vi "zero_detection_simulation.vi"() -> ()   [LabVIEW 2021]
uses:
  <vilib>/Platform/TimedLoop/XDataNode/timing_clust.ctl
  <vilib>/Platform/TimedLoop/XDataNode/nitl_modes.ctl
  <vilib>/Platform/TimedLoop/XDataNode/wakeup.ctl
  <vilib>/Platform/TimedLoop/XDataNode/XDataNode.xnode
  <vilib>/Platform/TimedLoop/XDataNode/XDNodeRunTimeDep.lvlib
panel:
  in  "stop 2":bool
  out "output":dbl(slide) scale=-1.0..1.0
  in  "fractional index or x":dbl(slide) scale=0.0..1.0
  out "size(s)":i32
  in  "sin wave":dbl
  in  "memory down sampling rate":i32
  in  "zero detect down sampling rate":i32
  out "Waveform Graph":dbl[](graph)
  out "appended array":dbl[](array[numeric])
  out "Disturbance(x)":dbl(graph)
  in  "stop":bool
  # "Disturbance"
  # "Online Segmentaion"
  # "Phase"
  # "Memory"
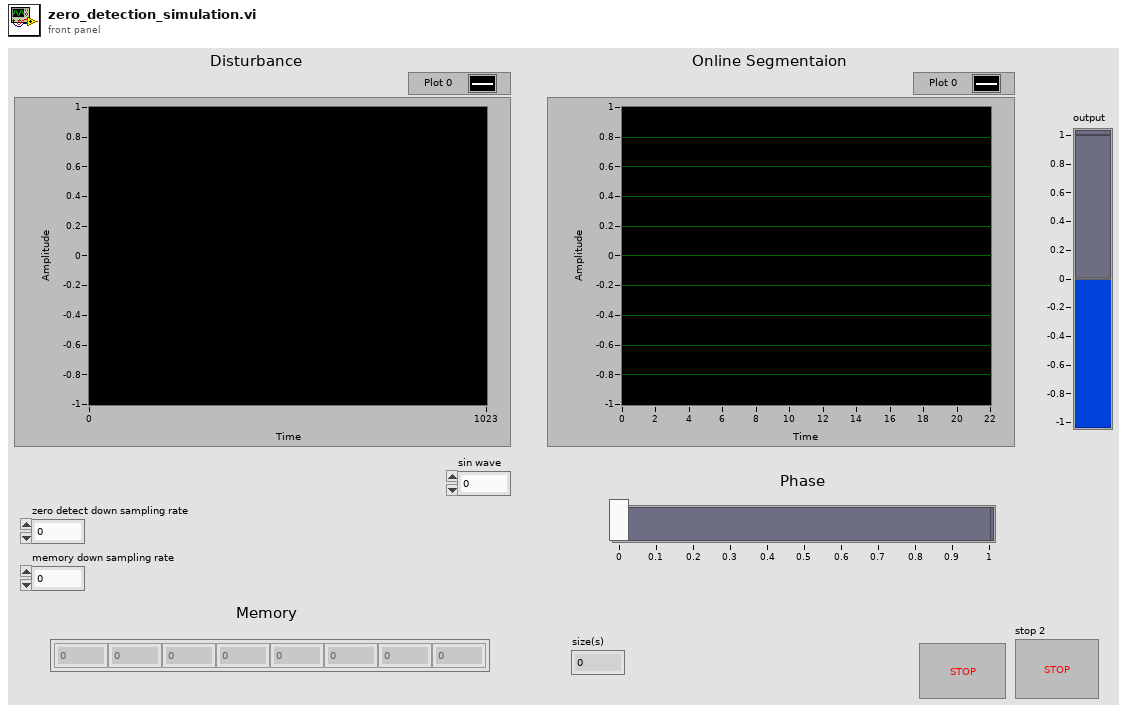
[diagram p1: front panel]
types:
  T1 = typedef "XDNodeRunTimeDep.lvlib/timing_clust.ctl" = cluster{"Expected End [f-1]":u64, "Actual End [f-1]":u64, "Finished Late? [f-1]":bool, "Expected End [i-1]":u64, "Actual End [i-1]":u64, "Finished Late? [i-1]":bool, "Expected Start [i]":u64, "Actual Start [i]":u64, "Expected Start [f]":u64, "Actual Start [f]":u64, "Source Name":string, "Structure Name":string, "Period":i64, "Deadline":i64, "Offset":i64, "Start":i64, "Priority":i32, "Timeout":i32, "Mode":T2, "Wakeup Reason":T3, "Error":errorcluster, "Source Type":string, "Secondary Source Type":string, "Global End Time":u64, "Global Start Time":u64, "Frame Duration":u64, "Iteration Duration":u64, "Assigned CPU":i32, "I/O Scan Engine Mode":u32}
  T2 = typedef "XDNodeRunTimeDep.lvlib/nitl_modes.ctl" = enum32{"No Change", "Process missed periods, maintain original phase", "Discard missed periods, maintain original phase", "Process missed periods, ignore original phase", "Discard missed periods, ignore original phase"}
  T3 = typedef "XDNodeRunTimeDep.lvlib/wakeup.ctl" = enum32{"Normal", "Aborted", "Asynchronous wakeup", "Timing source error", "Timed loop error", "Timeout"}
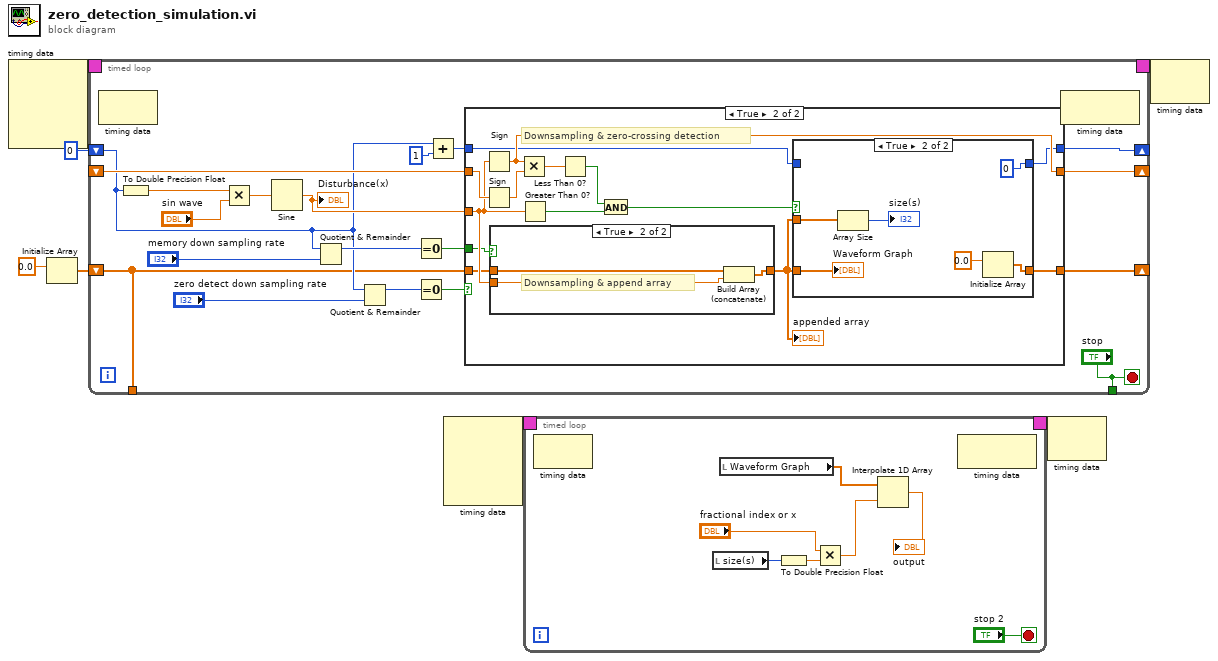
[diagram p0: block diagram]
diagram:
  n1 = node-c288() -> (w4:T1)  [unwired: 4 in]
  n2 = Initialize Array(0.0 ("element")) -> (w5:dbl[])  [unwired: 1 in]
  n3 = timed-loop {
    shift-right: [w23] -> _
    shift-left: _ -> [w22]
    shift-right: [w10] -> _
    shift-left: w5 -> [w9]
    shift-right: [w15] -> _
    shift-left: 0 -> [w16]
    timing: w4 -> [_]
    timing-out: [_] -> w3
    tunnel: [w9] -> _
    tunnel: ["stop"] -> _
    stop <- "stop" stop-if-true
    n4 = node-c288() -> ()  [unwired: 1 in, 1 out]
    n5 = To Double Precision Float(number=w16) -> (double precision float=w26:dbl)
    n6 = Multiply(x=w26, y="sin wave") -> (x*y=w21:dbl)
    n7 = Sine(x=w21) -> (sin(x)=w20:dbl)
    "Disturbance(x)" <- w20
    n8 = Quotient & Remainder(x=w16, y="memory down sampling rate") -> (x-y*floor(x/y)=w19:i32)  [unwired: 1 out]
    n9 = Quotient & Remainder(x=w16, y="zero detect down sampling rate") -> (x-y*floor(x/y)=w25:i32)  [unwired: 1 out]
    n10 = Equal To 0?(x=w19) -> (x = 0?=w18:bool)
    n11 = Equal To 0?(x=w25) -> (x = 0?=w24:bool)
    n12 = Add(x=w16, y=1) -> (x+y=w14:i32)
    n13 = case shown="True" w24 {
      tunnel: w20 -> [_ w40]
      tunnel: [w31 w43] -> w23
      tunnel: w22 -> [w31 w42]
      tunnel: [w30 w41] -> w10
      tunnel: w9 -> [w30 w34]
      tunnel: w18 -> [_ w32]
      tunnel: [w29 w36] -> w15
      tunnel: w14 -> [w29 w35]
      frame False {
      }
      frame True {
        # "Downsampling & zero-crossing detection"
        n14 = Sign(1:w40) -> (0:w43:dbl)
        n15 = Sign(1:w42) -> (0:w44:dbl)
        n16 = case shown="True" w32 {
          tunnel: w34 -> [w46 w49]
          tunnel: [w46 w48] -> w33
          tunnel: w40 -> [_ w47]
          frame False {
          }
          frame True {
            # "Downsampling & append array"
            n17 = Build Array (concatenate)(w49, w47) -> (w48:dbl[])
          }
        }
        "appended array" <- w33
        n18 = Multiply(x=w43, y=w44) -> (x*y=w45:dbl)
        n19 = Greater Than 0?(x=w40) -> (x > 0?=w38:bool)
        n20 = Less Than 0?(x=w45) -> (x < 0?=w39:bool)
        n21 = And(x=w39, y=w38) -> (x .and. y?=w37:bool)
        n22 = case shown="True" w37 {
          tunnel: w33 -> [w50 w52]
          tunnel: [w50 w57] -> w41
          tunnel: [w51 0] -> w36
          tunnel: w35 -> [w51 _]
          tunnel: w33 -> [_ w54]
          frame False {
          }
          frame True {
            n23 = Array Size(array=w54) -> (size(s)=→"size(s)":i32)
            n24 = Initialize Array(0.0 ("element")) -> (w57:dbl[])  [unwired: 1 in]
            "Waveform Graph" <- w52
          }
        }
      }
    }
    n25 = node-c288() -> ()  [unwired: 1 in, 1 out]
  }
  n26 = node-c288() -> (w2:T1)  [unwired: 4 in]
  n27 = timed-loop {
    timing: w2 -> [_]
    timing-out: [_] -> w1
    stop <- "stop 2" stop-if-true
    n28 = node-c288() -> ()  [unwired: 1 in, 1 out]
    n29 = local read "size(s)"() -> (w60:i32)
    n30 = local read "Waveform Graph"() -> (w59:dbl[])
    n31 = To Double Precision Float(number=w60) -> (double precision float=w63:dbl)
    n32 = Multiply(x="fractional index or x", y=w63) -> (x*y=w64:dbl)
    n33 = Interpolate 1D Array(1:w64, 2:w59) -> (0:→"output":dbl)
    n34 = node-c288() -> ()  [unwired: 1 in, 1 out]
  }
  n35 = node-c288(w1) -> ()  [unwired: 1 out]
  n36 = node-c288(w3) -> ()  [unwired: 1 out]
